vi "PC Reader.vi"(8 "error in (no error)":errorcluster, 10 "Photon Counter SR400 in":refnum<class "Photon Counter SR400.lvclass">, 11 "PC Reader in":refnum<class "PC Reader.lvclass">) -> (0 "error out":errorcluster, 3 "PC Reader out":refnum<class "PC Reader.lvclass">)   [LabVIEW 2017, in "PC Reader.lvclass"]
uses:
  PC Reader.lvclass
  C:/LabVIEW-programs-dev/Readers/Reader/Reader.lvclass
  Instruments/Photon Counter/Photon Counter SR400.lvclass
  C:/LabVIEW-programs-dev/Instruments/Utility Classes/Readable/Readable.lvclass
  Reader/Reader.lvclass
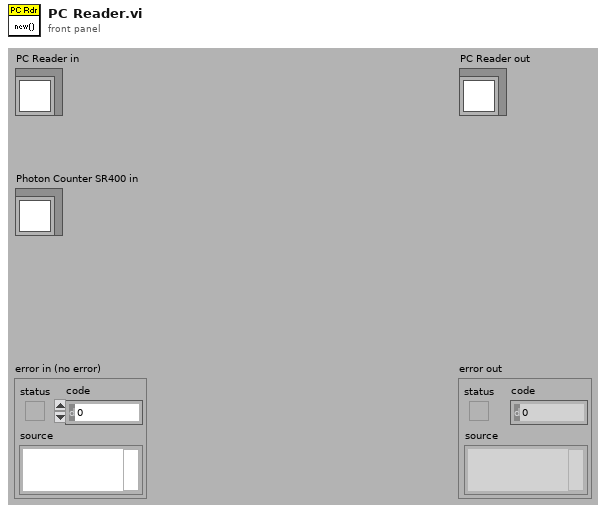
[diagram p1: front panel]
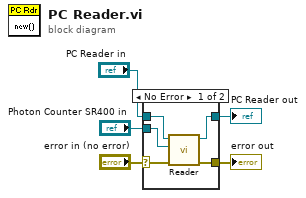
[diagram p0: block diagram]
diagram:
  n1 = case shown="No Error" "error in (no error)" {
    selector: "error in (no error)" -> [w9 w12]
    tunnel: [w8 w12] -> w4
    tunnel: [w6 w11] -> w2
    tunnel: "PC Reader in" -> [w10 w11]
    tunnel: "Photon Counter SR400 in" -> [w7 _]
    frame No Error {
      n2 = call "Reader.vi"("error in (no error)"=w9, "Readable"=w7, "Reader in"=w10) -> ("error out"=w8:errorcluster, "Reader out"=w6:refnum<class "PC Reader.lvclass">)  [unwired: 7 out]
    }
    frame Error {
    }
  }
  "error out" <- w4
  "PC Reader out" <- w2
